vi "SQL_test_template_insert.vi"(10 "表格控件":string[][](table), 11 "模板名称":string) -> (3 "error out":errorcluster)   [LabVIEW 2014]
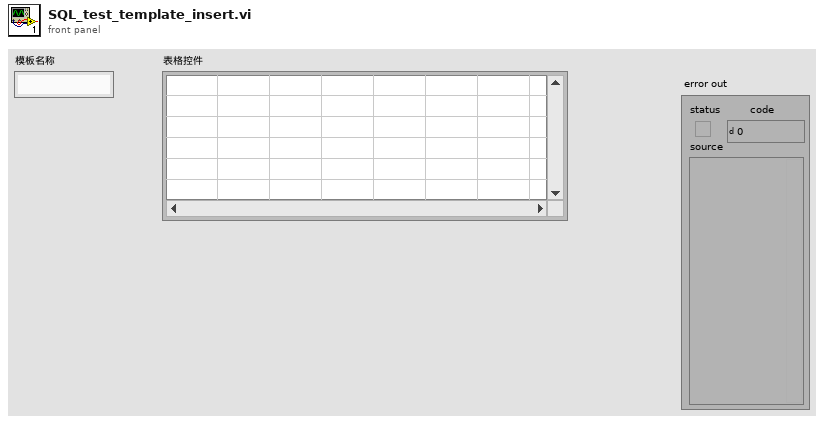
[diagram p1: front panel]
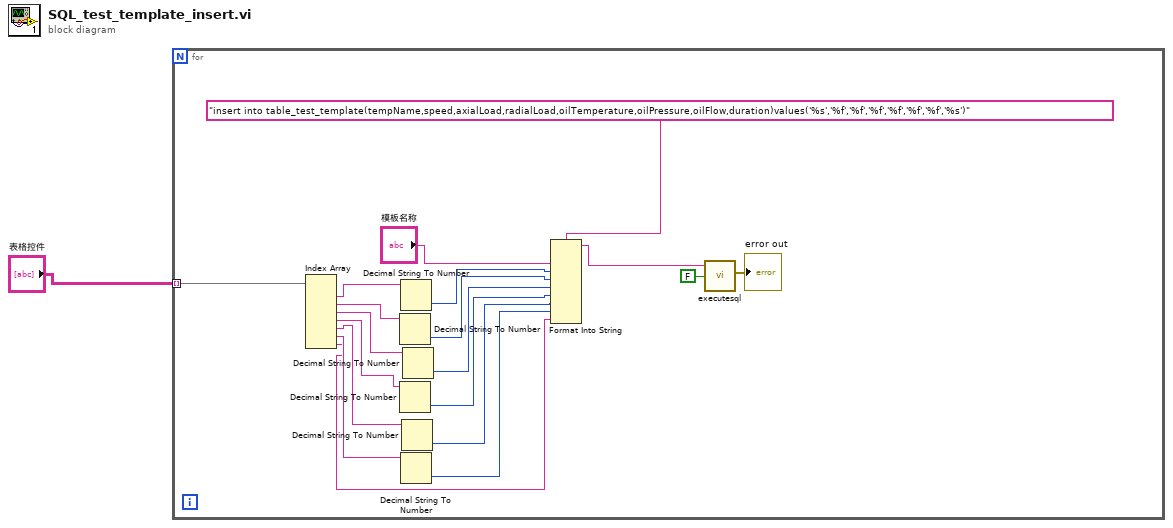
[diagram p0: block diagram]
diagram:
  n1 = for {
    tunnel: "表格控件" -> [w18] mode=indexing
    n2 = Index Array(array=w18) -> (element #1=w17:string, element #2=w15:string, element #3=w13:string, element #4=w11:string, element #5=w9:string, element #6=w7:string, element #7=w5:string)  [unwired: 7 in]
    n3 = Decimal String To Number(string=w15) -> (number=w14:i32)  [unwired: 2 in, 1 out]
    n4 = Decimal String To Number(string=w11) -> (number=w10:i32)  [unwired: 2 in, 1 out]
    n5 = Decimal String To Number(string=w17) -> (number=w16:i32)  [unwired: 2 in, 1 out]
    n6 = Decimal String To Number(string=w7) -> (number=w6:i32)  [unwired: 2 in, 1 out]
    n7 = Decimal String To Number(string=w9) -> (number=w8:i32)  [unwired: 2 in, 1 out]
    n8 = Decimal String To Number(string=w13) -> (number=w12:i32)  [unwired: 2 in, 1 out]
    n9 = Format Into String(format string="insert into table_test_template(tempName,speed,axialLoad,radialLoad,oilTemperature,oilPressure,oilFlow,duration)values('%s','%f','%f','%f','%f','%f','%f','%s')", "模板名称", w16, w14, w12, w10, w8, w6, w5) -> (resulting string=w4:string)  [unwired: 2 in, 1 out]
    n10 = call "executesql.vi"("Return Data (T)"=FALSE, "Command Text"=w4) -> ("error out"=→"error out":errorcluster)  [unwired: 5 in, 1 out]
  }
